vi "create_shared_link-with_settings.vi"(8 "error in (no error)":errorcluster) -> (0 "error out":errorcluster)   [LabVIEW 2015, in "lv-dropbox.lvlib" / "v2.lvlib"]
uses:
  v2.lvlib
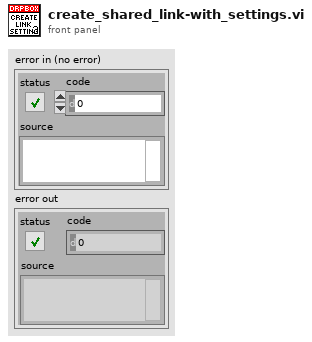
[diagram p1: front panel]
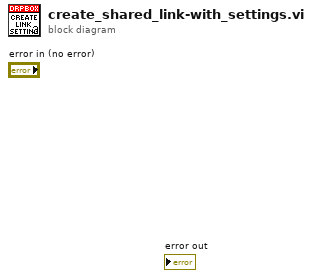
[diagram p0: block diagram]
diagram:
